vi "rs3_stop_process.vi"(9 "STOP and EXIT":bool, 11 "error in (no error)":errorcluster) -> ()   [LabVIEW 2019, in "libRealSense3.lvlib"]
doc: "It is important to close everything properly at the end. Use this VI to clean up and close the RealSense device, queue, sensor, and device list."
uses:
  libRealSense3.lvlib
panel:
  out "Standard error output":string
  out "Current Folder Path":path
  out "Current .vi file path":path
  out "Standard  output":string
  # "RS3 Stop Process"
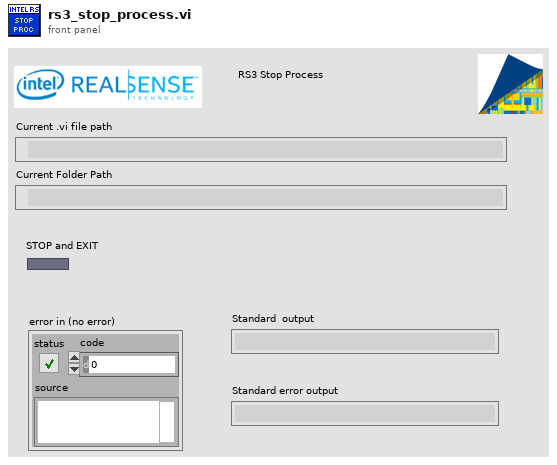
[diagram p1: front panel]
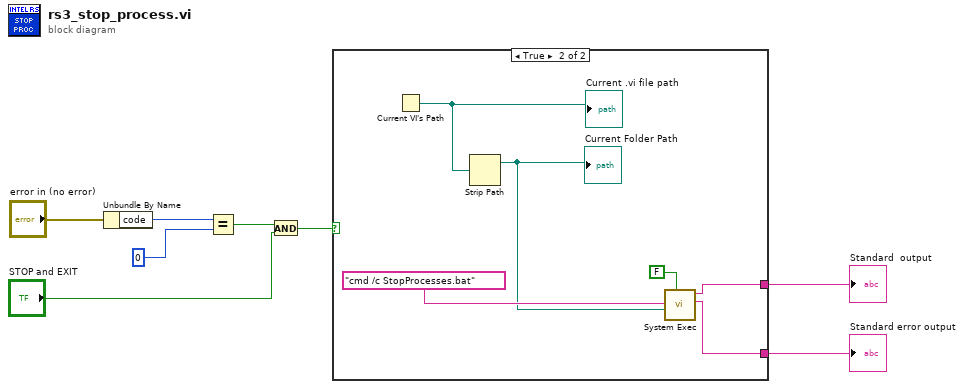
[diagram p0: block diagram]
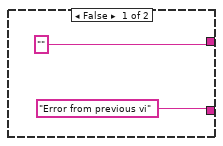
[diagram p2: hidden frame]
diagram:
  n1 = Unbundle By Name("error in (no error)") -> ("code"=w5:i32)
  n2 = Equal?(x=w5, y=0) -> (x = y?=w1:bool)
  n3 = And(x=w1, y="STOP and EXIT") -> (x .and. y?=w3:bool)
  n4 = case shown="True" w3 {
    tunnel: ["" w12] -> w8
    tunnel: ["Error from previous vi" w11] -> w7
    frame False {
    }
    frame True {
      n5 = Current VI's Path() -> (path=w16:path)
      "Current .vi file path" <- w16
      n6 = Strip Path(path=w16) -> (stripped path=w14:path)  [unwired: 1 out]
      "Current Folder Path" <- w14
      n7 = call <vilib>:"System Exec.vi"("wait until completion? (T)"=FALSE, "working directory"=w14, "command line"="cmd /c StopProcesses.bat") -> ("standard error"=w11:string, "standard output"=w12:string)  [unwired: 5 in, 2 out]
    }
  }
  "Standard  output" <- w8
  "Standard error output" <- w7
